vi "Resistance Test_BU2.vi"(0 "DMM ref in":refnum<visa-resource-name>, 2 "Resistance Test REF":refnum<vi>, 3 "Resistance Test Stop REF":refnum<vi>, 5 "DMM error in":errorcluster, 7 "Channel  Count":i32, 9 "ESP32 ref in":refnum<visa-resource-name>="COM4", 11 "ESP32 error in":errorcluster, 12 "Wait Current Stable Period":u32, 14 "Current Sense \nResitance Array":dbl[](array[numeric])) -> (1 "Array 2":bool[](array[boolean]), 6 "error?":bool, 8 "Array":dbl[](array[numeric]), 10 "ESP32 ref out":refnum<visa-resource-name>, 15 "ESP32 error out":errorcluster)   [LabVIEW 2023]
uses:
  <instrlib>/Agilent 3446X Series/Agilent 3446X Series.lvlib
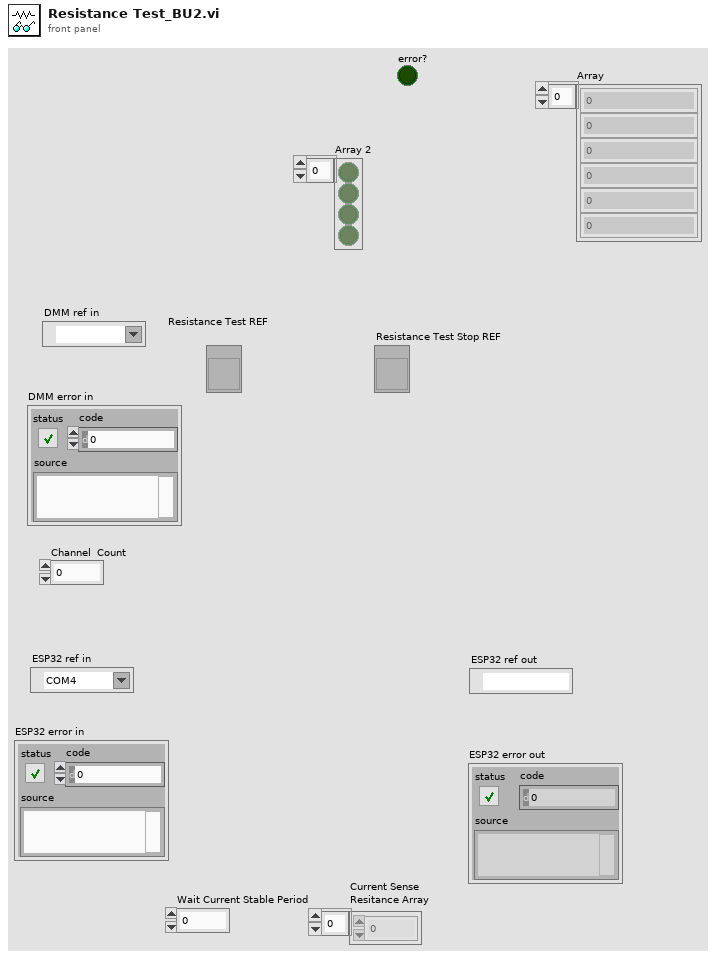
[diagram p1: front panel]
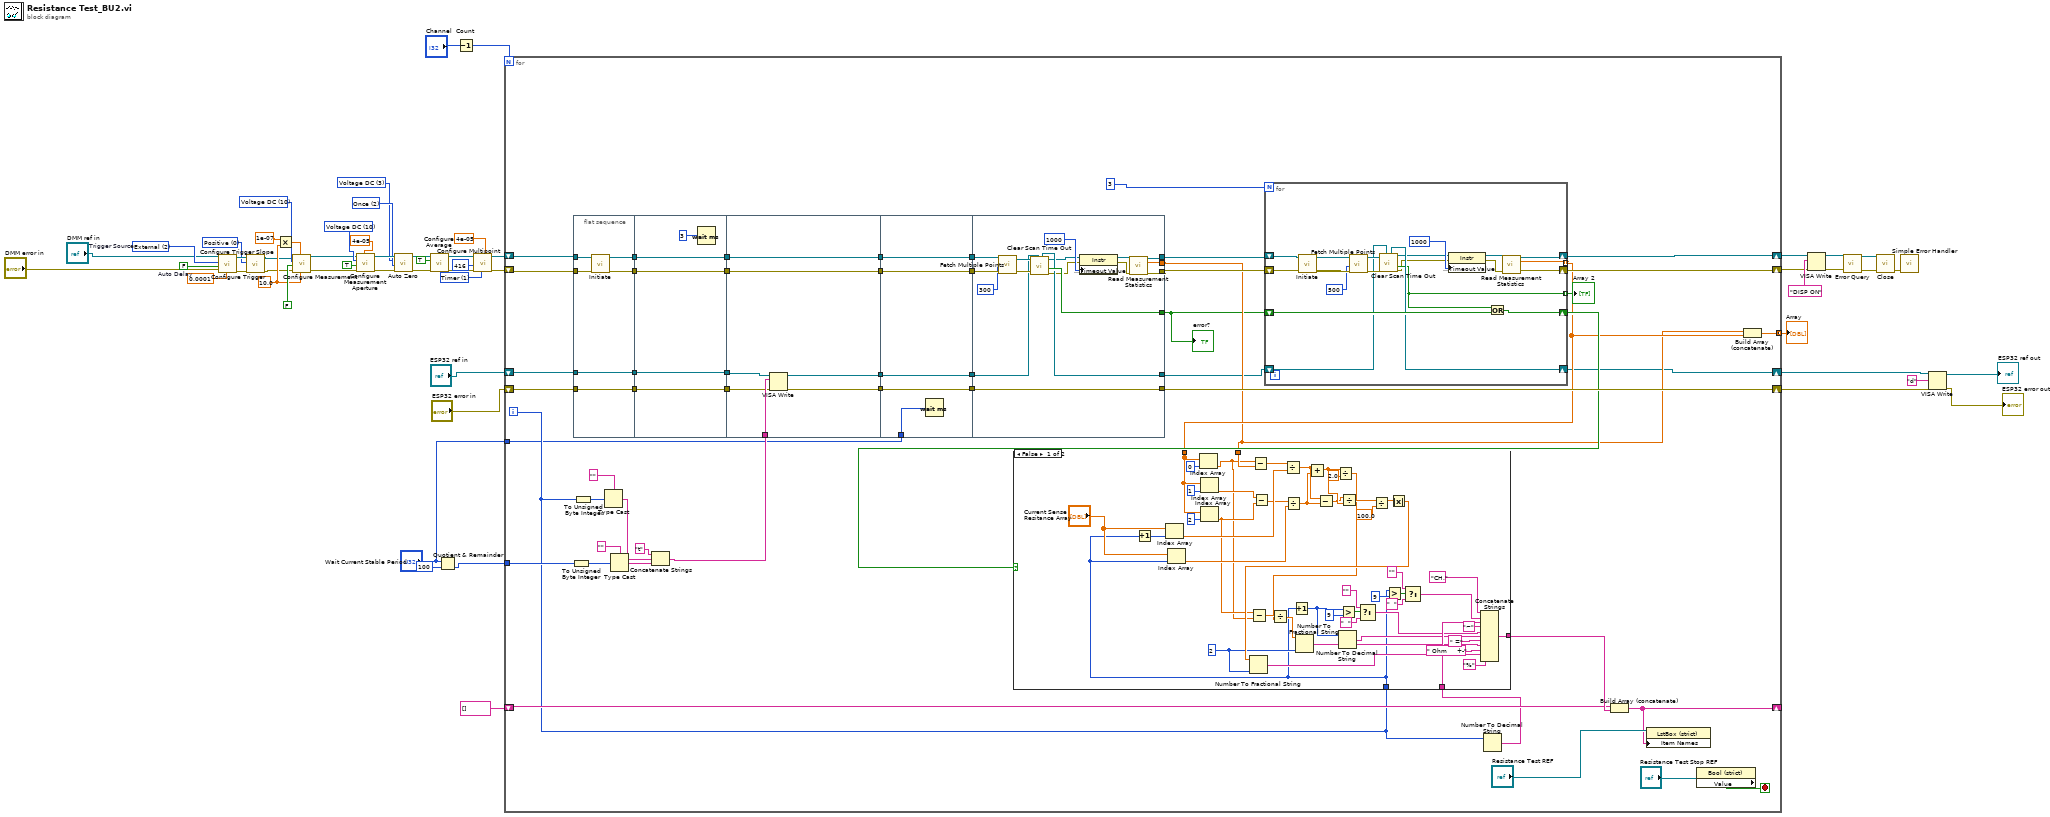
[diagram p0: block diagram]
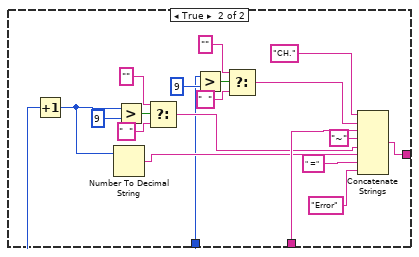
[diagram p2: hidden frame]
diagram:
  w16 = 0 items=["Positive", "Negative"] ("Trigger Edge (1: Negative)")
  w14 = 2 items=["Immediate", "Software (Bus)", "External"]  # Trigger Source
  w15 = FALSE  # Auto Delay
  w19 = 10.0 ("Manual Range (1)")
  w23 = 10 items=["Continuity", "Current AC", "Current DC", "Diode", "Frequency", "Resistance 4-wire", "Period", "Resistance 2-wire", "Temperature", "Voltage AC", "Voltage DC", "Voltage DC Ratio", "Capacitance"] ("Measurement Function (10: Voltage DC)")
  w27 = 1 items=["Immediate", "Timer"] ("Sample Source (0: Immediate)")
  w34 = 3 items=["Current DC", "Resistance", "Temperature", "Voltage DC"] ("Zero Type (0: Current DC)")
  w35 = 2 items=["Disable", "Enable", "Once"] ("Auto Zero (1: Enable)")
  w31 = 10 items=["Continuity", "Current AC", "Current DC", "Diode", "Frequency", "Resistance 4-wire", "Period", "Resistance 2-wire", "Temperature", "Voltage AC", "Voltage DC", "Voltage DC Ratio", "Capacitance"] ("Measurement Function (0: Continuity)")
  n1 = call <instrlib>:"Configure Trigger.vi"("Manual Trigger Delay (1 s)"=0.0001, "error in (no error)"="DMM error in", "Auto Delay (F:Disable)"=w15, "Trigger Source (0: Immediate)"=w14, "VISA resource name"="DMM ref in") -> ("error out"=w18:errorcluster, "VISA resource name out"=w17:refnum<visa-resource-name>)  [unwired: 1 in, 4 out]
  n2 = call <instrlib>:"Configure Trigger Slope.vi"("error in (no error)"=w18, "Trigger Edge (1: Negative)"=w16, "VISA resource name"=w17) -> ("error out"=w11:errorcluster, "VISA resource name out"=w12:refnum<visa-resource-name>)  [unwired: 7 in]
  n3 = Multiply(x=1e-07, y=w19) -> (x*y=w24:dbl)
  n4 = call <instrlib>:"Configure Measurement.vi"("Manual Range (1)"=w19, "Absolute Resolution (1E-6)"=w24, "error in (no error)"=w11, "Auto Range (T: Enable)"=FALSE, "Measurement Function (10: Voltage DC)"=w23, "VISA resource name"=w12) -> ("error out"=w20:errorcluster, "VISA resource name out"=w21:refnum<visa-resource-name>)  [unwired: 4 out]
  n5 = call <instrlib>:"Configure Measurement Aperture.vi"("Aperture Time (0.1s)"=4e-05, "error in (no error)"=w20, "Enable Aperture (F: Disable)"=TRUE, "Measurement Function (0: Continuity)"=w31, "VISA resource name"=w21) -> ("error out"=w38:errorcluster, "VISA resource name out"=w37:refnum<visa-resource-name>)  [unwired: 5 in]
  n6 = call <instrlib>:"Auto Zero.vi"("error in (no error)"=w38, "Auto Zero (1: Enable)"=w35, "Zero Type (0: Current DC)"=w34, "VISA resource name"=w37) -> ("error out"=w40:errorcluster, "VISA resource name out"=w39:refnum<visa-resource-name>)  [unwired: 6 in]
  n7 = call <instrlib>:"Configure Average.vi"("error in (no error)"=w40, "Enable Statistics (F: Disable)"=TRUE, "VISA resource name"=w39) -> ("error out"=w29:errorcluster, "VISA resource name out"=w30:refnum<visa-resource-name>)  [unwired: 7 in]
  n8 = Quotient & Remainder(x="Wait Current Stable Period", y=100) -> (floor(x/y)=w5:u32)  [unwired: 1 out]
  n9 = Decrement(x="Channel  Count") -> (x-1=w3:i32)
  n10 = call <instrlib>:"Configure Multipoint.vi"("Sample Interval (1 Second)"=4e-05, "Sample Source (0: Immediate)"=w27, "error in (no error)"=w29, "Sample Count (1)"=416, "VISA resource name"=w30) -> ("error out"=w9:errorcluster, "VISA resource name out"=w10:refnum<visa-resource-name>)  [unwired: 2 in, 3 out]
  n11 = for {
    N: w3 -> [_]
    shift-right: [w66] -> w42
    shift-left: "ESP32 ref in" -> [w90]
    shift-right: [w76] -> w4
    shift-left: "ESP32 error in" -> [w88]
    shift-right: [w100] -> w43
    shift-left: w9 -> [w94]
    shift-right: [w101] -> w44
    shift-left: w10 -> [w95]
    shift-right: [w103] -> _
    shift-left: string[] [] -> [w105]
    tunnel: w5 -> [w78]
    tunnel: [w70] -> w2 mode=concatenating
    tunnel: "Wait Current Stable Period" -> [w57]
    i -> [w74]
    stop <- w107 stop-if-true
    n12 = To Unsigned Byte Integer(number=w78) -> (unsigned 8bit integer=w82:u8)
    n13 = flat-sequence {
      tunnel: w94 -> [w180]
      tunnel: w95 -> [w182]
      tunnel: [w181] -> w99
      tunnel: [w179] -> w98
      tunnel: [w178] -> w91
      tunnel: w90 -> [w178]
      tunnel: w88 -> [w177]
      tunnel: [w177] -> w87
      tunnel: [w187] -> w97
      tunnel: [w186] -> w96
      tunnel: w99 -> [w187]
      tunnel: w98 -> [w186]
      tunnel: w91 -> [w184]
      tunnel: [w184] -> w89
      tunnel: w87 -> [w183]
      tunnel: [w183] -> w86
      tunnel: w97 -> [w194]
      tunnel: [w194] -> w63
      tunnel: w96 -> [w193]
      tunnel: [w193] -> w65
      tunnel: w89 -> [w192]
      tunnel: w86 -> [w190]
      tunnel: w77 -> [w191]
      tunnel: [w189] -> w61
      tunnel: [w188] -> w59
      tunnel: w65 -> [w199]
      tunnel: [w199] -> w64
      tunnel: w63 -> [w198]
      tunnel: [w198] -> w62
      tunnel: w61 -> [w197]
      tunnel: [w197] -> w60
      tunnel: w59 -> [w196]
      tunnel: [w196] -> w58
      tunnel: w57 -> [w195]
      tunnel: [w213] -> w92
      tunnel: [w214] -> w93
      tunnel: w64 -> [w216]
      tunnel: w62 -> [w215]
      tunnel: [w205] -> w67
      tunnel: w60 -> [w207]
      tunnel: [w211] -> w76
      tunnel: w58 -> [w211]
      tunnel: [w210] -> w71
      tunnel: [w206] -> w68
      frame #0 {
        n14 = call <instrlib>:"Initiate.vi"("error in (no error)"=w180, "VISA resource name"=w182) -> ("error out"=w179:errorcluster, "VISA resource name out"=w181:refnum<visa-resource-name>)  [unwired: 8 out]
      }
      frame #1 {
        n15 = Wait (ms)(milliseconds to wait=u32 3) -> ()  [unwired: 1 out]
      }
      frame #2 {
        n16 = VISA Write(VISA resource name=w192, write buffer=w191, error in (no error)=w190) -> (VISA resource name out=w189:refnum<visa-resource-name>, error out=w188:errorcluster)  [unwired: 1 out]
      }
      frame #3 {
        n17 = Wait (ms)(milliseconds to wait=w195) -> ()  [unwired: 1 out]
      }
      frame #4 {
        n18 = call <instrlib>:"Fetch Multiple Points.vi"("error in (no error)"=w216, "Timeout (10000 ms)"=300, "VISA resource name"=w215) -> ("error out"=w208:errorcluster, "VISA resource name out"=w209:refnum<visa-resource-name>)  [unwired: 1 in, 6 out]
        n19 = call "Clear Scan Time Out.vi"("ESP32 ref"=w207, "error in (no error)"=w208, "VISA Refnum in"=w209) -> ("error out"=w202:errorcluster, "error?"=w206:bool, "VISA Refnum out"=w203:refnum<visa-resource-name>, "ESP32 ref out"=w205:refnum<visa-resource-name>)  [unwired: 4 in, 1 out]
        n20 = property class="Instr"(reference=w203, error in=w202, "General Settings:Timeout Value"=u32 1000) -> (reference out=w201:refnum<visa-resource-name>, error out=w200:errorcluster)
        n21 = call <instrlib>:"Read Measurement Statistics.vi"("VISA resource name"=w201, "error in (no error)"=w200) -> ("VISA resource name out"=w214:refnum<visa-resource-name>, "Arithmetic Mean"=w210:dbl, "error out"=w213:errorcluster)  [unwired: 6 in, 5 out]
      }
    }
    n22 = To Unsigned Byte Integer(number=w74) -> (unsigned 8bit integer=w79:u8)
    n23 = Type Cast(type="" ("string"), x=w79) -> (*(type *) &x=w80:string)
    n24 = Type Cast(type="" ("string"), x=w82) -> (*(type *) &x=w81:string)
    n25 = Concatenate Strings("t" ("data in"), w80, w81) -> (w77:string)
    n26 = for {
      N: 3 -> [_]
      tunnel: [w232] -> w72 mode=indexing
      shift-right: [w230] -> w101
      shift-left: w93 -> [w234]
      shift-right: [w229] -> w100
      shift-left: w92 -> [w233]
      shift-right: [w227] -> w73
      shift-left: w68 -> [w228]
      tunnel: [w222] -> w69 mode=indexing
      shift-right: [w223] -> w66
      shift-left: w67 -> [w224]
      n27 = call <instrlib>:"Initiate.vi"("error in (no error)"=w233, "VISA resource name"=w234) -> ("error out"=w236:errorcluster, "VISA resource name out"=w235:refnum<visa-resource-name>)  [unwired: 8 out]
      n28 = call <instrlib>:"Fetch Multiple Points.vi"("error in (no error)"=w236, "Timeout (10000 ms)"=500, "VISA resource name"=w235) -> ("error out"=w225:errorcluster, "VISA resource name out"=w226:refnum<visa-resource-name>)  [unwired: 1 in, 6 out]
      n29 = call "Clear Scan Time Out.vi"("ESP32 ref"=w224, "error in (no error)"=w225, "VISA Refnum in"=w226) -> ("error out"=w217:errorcluster, "error?"=w222:bool, "VISA Refnum out"=w218:refnum<visa-resource-name>, "ESP32 ref out"=w223:refnum<visa-resource-name>)  [unwired: 4 in, 1 out]
      n30 = property class="Instr"(reference=w218, error in=w217, "General Settings:Timeout Value"=u32 1000) -> (reference out=w220:refnum<visa-resource-name>, error out=w219:errorcluster)
      n31 = Or(x=w222, y=w228) -> (x .or. y?=w227:bool)
      n32 = call <instrlib>:"Read Measurement Statistics.vi"("VISA resource name"=w220, "error in (no error)"=w219) -> ("VISA resource name out"=w230:refnum<visa-resource-name>, "Arithmetic Mean"=w232:dbl, "error out"=w229:errorcluster)  [unwired: 6 in, 5 out]
    }
    "Array 2" <- w69
    n33 = Number To Decimal String(number=w74) -> (decimal integer string=w75:string)  [unwired: 1 in]
    n34 = case shown="False" w73 {
      tunnel: [w152 w171] -> w106
      tunnel: w75 -> [w149 w168]
      tunnel: w72 -> [w137 _]
      tunnel: w74 -> [w113 w159]
      tunnel: w71 -> [w130 _]
      frame False {
        w121 = i16 2 ("precision (6)")
        n35 = Increment(x=w113) -> (x+1=w133:i32)
        n36 = Index Array(array="Current Sense \nResitance Array", index=w133) -> (element=w131:dbl)
        n37 = Index Array(array="Current Sense \nResitance Array", index=w113) -> (element=w128:dbl)
        n38 = Index Array(array=w137, index=0) -> (element=w117:dbl)
        n39 = Index Array(array=w137, index=1) -> (element=w118:dbl)
        n40 = Index Array(array=w137, index=2) -> (element=w119:dbl)
        n41 = Subtract(x=w119, y=w117) -> (x-y=w116:dbl)
        n42 = Subtract(x=w117, y=w130) -> (x-y=w134:dbl)
        n43 = Subtract(x=w118, y=w119) -> (x-y=w129:dbl)
        n44 = Divide(x=w134, y=w131) -> (x/y=w126:dbl)
        n45 = Divide(x=w129, y=w128) -> (x/y=w125:dbl)
        n46 = Increment(x=w113) -> (x+1=w142:i32)
        n47 = Add(x=w126, y=w125) -> (x+y=w112:dbl)
        n48 = Subtract(x=w126, y=w125) -> (x-y=w111:dbl)
        n49 = Divide(x=w112, y=2.0) -> (x/y=w115:dbl)
        n50 = Divide(x=w116, y=w115) -> (x/y=w114:dbl)
        n51 = Number To Fractional String(number=w114, precision (6)=w121) -> (F-format string=w123:string)  [unwired: 2 in]
        n52 = Number To Decimal String(number=w142) -> (decimal integer string=w141:string)  [unwired: 1 in]
        n53 = Greater?(x=w142, y=9) -> (0:w146:bool)
        n54 = Divide(x=w111, y=w112) -> (x/y=w124:dbl)
        n55 = Select(t="" ("string"), s=w146, f="  " ("string")) -> (s? t:f=w143:string)
        n56 = Divide(x=w124, y=100.0) -> (x/y=w110:dbl)
        n57 = Greater?(x=w113, y=9) -> (0:w155:bool)
        n58 = Absolute Value(x=w110) -> (abs(x)=w122:dbl)
        n59 = Number To Fractional String(number=w122, precision (6)=w121) -> (F-format string=w120:string)  [unwired: 2 in]
        n60 = Select(t="" ("string"), s=w155, f="  " ("string")) -> (s? t:f=w150:string)
        n61 = Concatenate Strings("CH." ("string"), w150, w149, "~" ("string"), w143, w141, " =" ("string"), w123, " Ohm     +-" ("string"), w120, "%" ("string")) -> (w152:string)
      }
      frame True {
        n62 = Increment(x=w159) -> (x+1=w161:i32)
        n63 = Number To Decimal String(number=w161) -> (decimal integer string=w160:string)  [unwired: 1 in]
        n64 = Greater?(x=w161, y=9) -> (0:w165:bool)
        n65 = Select(t="" ("string"), s=w165, f="  " ("string")) -> (s? t:f=w162:string)
        n66 = Greater?(x=w159, y=9) -> (0:w174:bool)
        n67 = Select(t="" ("string"), s=w174, f="  " ("string")) -> (s? t:f=w169:string)
        n68 = Concatenate Strings("CH." ("string"), w169, w168, "~" ("string"), w162, w160, " =" ("string"), "Error" ("string")) -> (w171:string)
      }
    }
    n69 = Build Array (concatenate)(w105, w106) -> (w103:string[])
    n70 = property class="LstBox (strict)"(reference="Resistance Test REF", "Item Names"=w103) -> ()  [unwired: 1 in, 2 out]
    n71 = property class="Bool (strict)"(reference="Resistance Test Stop REF") -> ("Value"=w107:bool)  [unwired: 1 in, 2 out]
    n72 = Build Array (concatenate)(w71, w72) -> (w70:dbl[])
    "error?" <- w68
  }
  "Array" <- w2
  n73 = VISA Write(VISA resource name=w44, write buffer="DISP ON", error in (no error)=w43) -> (VISA resource name out=w51:refnum<visa-resource-name>, error out=w50:errorcluster)  [unwired: 1 out]
  n74 = call <instrlib>:"Error Query.vi"("error in (no error)"=w50, "VISA resource name"=w51) -> ("error out"=w56:errorcluster, "VISA resource name out"=w55:refnum<visa-resource-name>)  [unwired: 8 out]
  n75 = call <instrlib>:"Close.vi"("error in (no error)"=w56, "VISA resource name"=w55) -> ("error out"=w54:errorcluster)  [unwired: 9 out]
  n76 = call <vilib>:"Simple Error Handler.vi"("error in (no error)"=w54) -> ()  [unwired: 1 in, 8 out]
  n77 = VISA Write(VISA resource name=w42, write buffer="d" ("data in"), error in (no error)=w4) -> (VISA resource name out=→"ESP32 ref out":refnum<visa-resource-name>, error out=→"ESP32 error out":errorcluster)  [unwired: 1 out]
